vi "HovaCAL fixed Komponents Formeln.vi"(8 "Fehler (Eingang)":errorcluster, 11 "Formel String in":string) -> (0 "Fehler (Ausgang)":errorcluster, 1 "HovaCAL fixed Formel Array":string[](array[string]), 2 "HovaCAL fixed Formel String":string, 3 "Formel String out":string, 5 "HovaCAL fixed":bool)   [LabVIEW 2020, in "Linearisierung v2.lvlib" / "SpanEinstellungen.lvlib"]
uses:
  SpanEinstellungen.lvlib
  Gasteiler/Aktion FGV Gasteilerliste laden.ctl
  Seiten/FT-IR/FGV FT-IR Gasliste Aktionen.ctl
  Gasteiler/Gasteiler.lvlib
  Seiten/FT-IR/FT-IR.lvlib
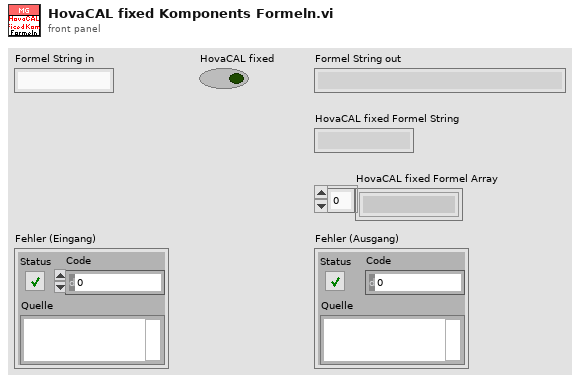
[diagram p1: front panel]
types:
  T1 = typedef "FT-IR.lvlib/FGV FT-IR Gasliste Aktionen.ctl" = enum16{"lesen", "Gasliste FT-IR", "Gasliste ausgelesen", "laden", "speichern", "löschen"}
  T2 = typedef "Linearisierung v2.lvlib/Gasteiler.lvlib/Aktion FGV Gasteilerliste laden.ctl" = enum16{"lesen", "laden", "speichern", "Liste erstellen", "Formel ändern", "Gas vereinzeln"}
  T3 = typedef "String - Ausgabefeld.ctl" = string
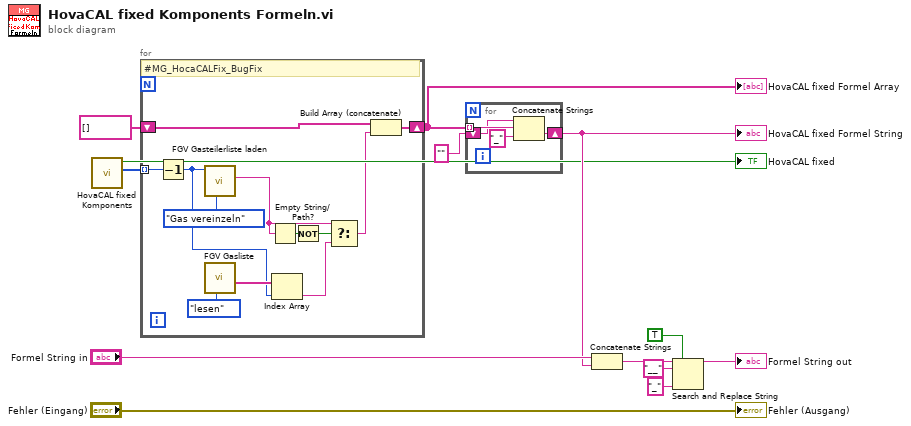
[diagram p0: block diagram]
diagram:
  n1 = call "HovaCAL fixed Komponents.vi"() -> ("MFV Komponente fix out"=w13:u16[], "HovaCAL fixed"=→"HovaCAL fixed":bool)  [unwired: 10 in]
  n2 = for {
    tunnel: w13 -> [w24] mode=indexing
    shift-right: [w23] -> w10
    shift-left: string[] [] -> [w22]
    # "#MG_HocaCALFix_BugFix"
    n3 = Decrement(x=w24) -> (x-1=w16:u16)
    n4 = call "FGV Gasteilerliste laden.vi"("Aktion"=Aktion_FGV_Gasteilerliste_laden."Gas vereinzeln", "Gasindex"=w16) -> ("Formel"=w17:string)  [unwired: 7 in, 2 out]
    n5 = call "FGV Gasliste.vi"("Aktionen"=FGV_FT-IR_Gasliste_Aktionen."lesen") -> ("Aktuelle Gasliste gesamt"=w19:T3[])  [unwired: 8 in, 2 out]
    n6 = Empty String/Path?(string/path=w17) -> (empty?=w20:bool)
    n7 = Index Array(array=w19, index=w16) -> (element=w21:T3)
    n8 = Not(x=w20) -> (.not. x?=w14:bool)
    n9 = Select(t=w17, s=w14, f=w21) -> (s? t:f=w15:T3)
    n10 = Build Array (concatenate)(w22, w15) -> (w23:T3[])
  }
  "HovaCAL fixed Formel Array" <- w10
  n11 = for {
    tunnel: w10 -> [w29] mode=indexing
    shift-right: [w26] -> w8
    shift-left: "" -> [w27]
    n12 = Concatenate Strings(w27, w29, "_") -> (w26:string)
  }
  "HovaCAL fixed Formel String" <- w8
  n13 = Concatenate Strings("Formel String in", w8) -> (w7:string)
  n14 = Search and Replace String(replace all?=TRUE ("Alle ersetzen? (F)"), input string=w7, search string="__" ("Such-String"), replace string="_" ("Ersetzungs-String (\"\")")) -> (result string=→"Formel String out":string)  [unwired: 4 in, 3 out]
  "Fehler (Ausgang)" <- "Fehler (Eingang)"
